vi "Ctx Term.vi"(7 "path override":path, 8 "error in (no error)":errorcluster, 11 "context_":u64) -> (0 "error out":errorcluster)   [LabVIEW 2025, in "libzmq-v143-mt-4_3_6.lvlib"]
doc: "ZMQ_EXPORT int zmq_ctx_term (void *context_);"
uses:
  libzmq-v143-mt-4_3_6.lvlib
  errno.vi
  strerror.vi
  <vilib>/Utility/error.llb/Error Cluster From Error Code.vi
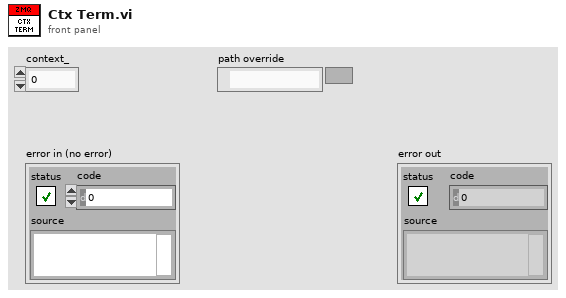
[diagram p1: front panel]
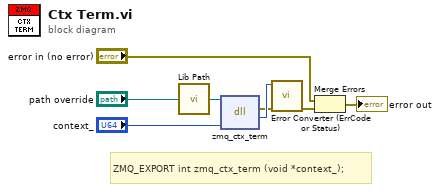
[diagram p0: block diagram]
diagram:
  # "ZMQ_EXPORT int zmq_ctx_term (void *context_);"
  n1 = call "Lib Path.vi"("path override"="path override") -> ("lib path"=w1:path)
  n2 = dll-call lib="home/james/Documents/ZeroMQ_LV/libzmq-v143-mt-4_3_6/libzmq.so" fn="zmq_ctx_term"(path in=w1, "context_"="context_") -> (error out=w6:errorcluster, "return type"=w8:i32)  [unwired: 3 in, 1 out]
  n3 = call "Error Converter (ErrCode or Status).vi"("error in (no error)"=w6, "error code"=w8) -> ("error out"=w5:errorcluster)  [unwired: 9 in]
  n4 = Merge Errors("error in (no error)", w5) -> (→"error out":errorcluster)
